vi "Scale Thumb.vi"(2 "Desired Dimensions":cluster{"Width":i32, "Height":i32}={"Width"=-1, "Height"=-1}, 3 "Full Size":bool=TRUE, 4 "Offset":cluster{"X":sgl, sgl}={"X"=-1.0, 0.0}, 5 "file":string, 6 "picture in":picture, 7 "Mod":T1) -> (0 "frame":T2, 1 "new picture":picture)   [LabVIEW 2012]
uses:
  SlideParams.ctl
  LVPresent_Globals.vi
panel:
  out "Dimensions":cluster{"Width":i32, "Height":i32}
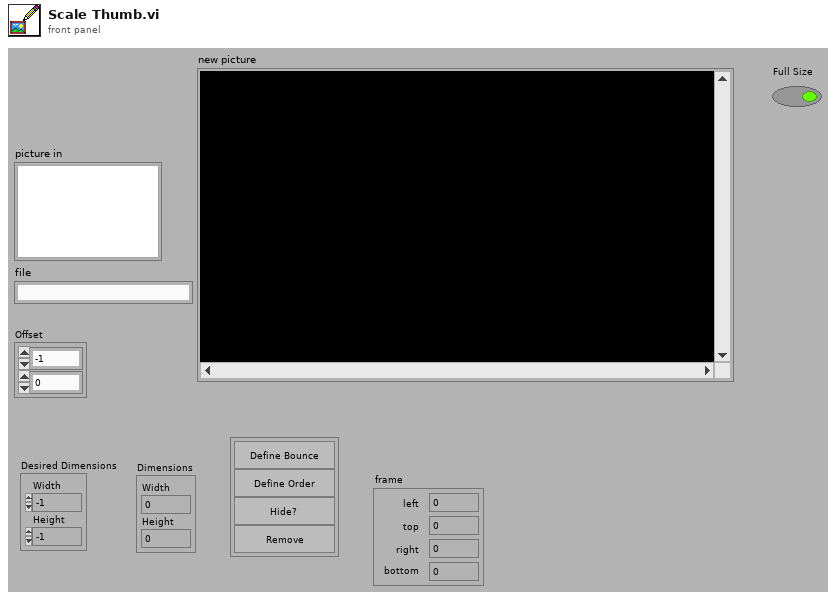
[diagram p1: front panel]
types:
  T1 = typedef "SlideParams.ctl" = enum32{"No Selection", "Bounce", "Order", "Hide", "Remove"}
  T2 = cluster{"left":i16, "top":i16, "right":i16, "bottom":i16}
  T3 = typedef "LVPositionTypeDef.ctl" = cluster{"Left":i32, "Top":i32}
  T4 = typedef "ParamterCluster.ctl" = cluster{"bounce?":bool, "black?":bool, "slide number":i32, "hide?":bool, "selection":bool}
  T5 = typedef "QT_Image.ctl" = cluster{"Width":i32, "Height":i32, "Depth":i32, "data":u8[], "Compressed data":u8[], "Color table":u32[], "Duration":i32, "Options":i32, "Timestamp":i32, "ID":i32, "Reserved":i32, "Dialogs":u32}
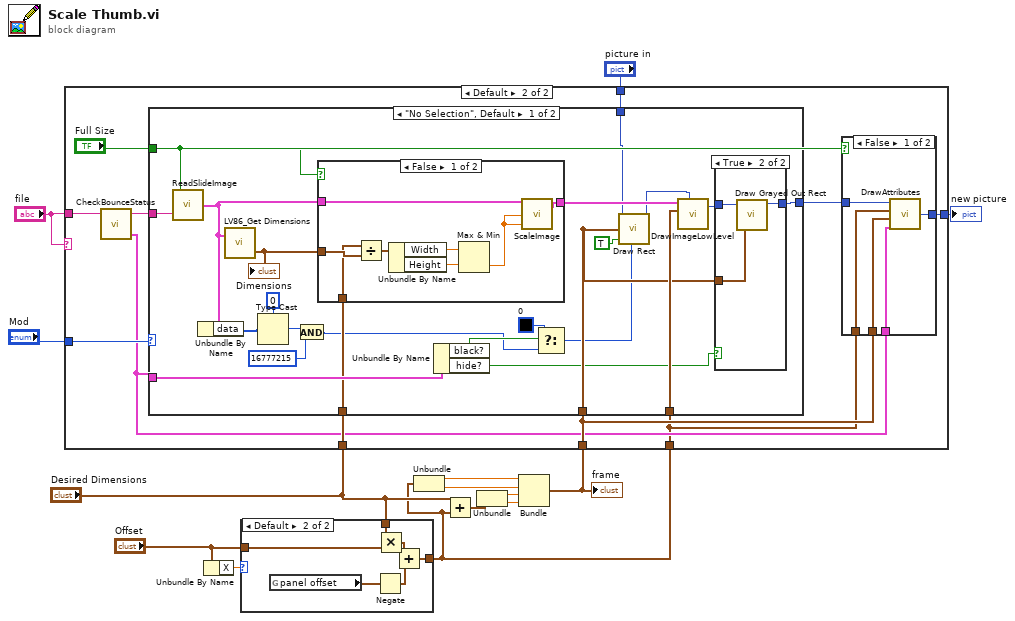
[diagram p0: block diagram]
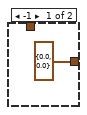
[diagram p2: hidden frame]
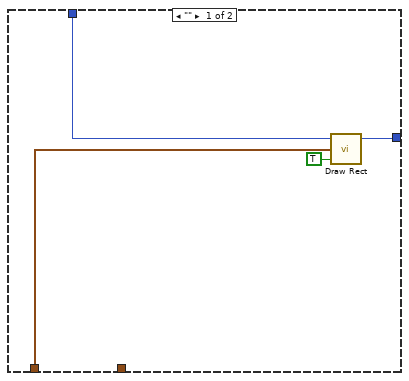
[diagram p3: hidden frame]
diagram:
  n1 = Unbundle By Name("Offset") -> ("X"=w1:sgl)
  n2 = case shown="Default" w1 {
    tunnel: "Desired Dimensions" -> [_ w20]
    tunnel: [cluster{sgl, sgl} {0.0, 0.0} w18] -> w3
    tunnel: "Offset" -> [_ w16]
    frame -1 {
    }
    frame Default {
      n3 = global read "LVPresent_Globals.vi" "panel offset"() -> (w17:T3)
      n4 = Negate(x=w17) -> (-x=w19:T3)
      n5 = Multiply(x=w20, y=w16) -> (x*y=w21:cluster{sgl, sgl})
      n6 = Add(x=w21, y=w19) -> (x+y=w18:cluster{sgl, sgl})
    }
  }
  n7 = Unbundle(w3) -> (w13:sgl, w12:sgl)
  n8 = Add(x="Desired Dimensions", y=w3) -> (x+y=w11:cluster{sgl, sgl})
  n9 = Unbundle(w11) -> (w10:sgl, w9:sgl)
  n10 = Bundle(w13, w12, w10, w9) -> (w7:cluster{sgl, sgl, sgl, sgl})  [unwired: 1 in]
  "frame" <- w7
  n11 = case shown="Default" "file" {
    tunnel: "picture in" -> [w25 w36]
    tunnel: "Desired Dimensions" -> [_ w35]
    tunnel: "file" -> [_ w33]
    tunnel: [w24 w31] -> w8
    tunnel: w7 -> [w23 w30]
    tunnel: w3 -> [_ w27]
    tunnel: "Mod" -> [_ w29]
    frame "" {
      n12 = call <vilib>:"Draw Rect.vi"("picture"=w25, "rect"=w23, "fill?(F)"=TRUE) -> ("new picture"=w24:picture)  [unwired: 6 in]
    }
    frame Default {
      n13 = call "CheckBounceStatus.vi"("File Name"=w33) -> ("Parameters"=w28:T4, "file name"=w34:string)  [unwired: 1 in, 1 out]
      n14 = case shown="\"No Selection\", Default" w29 {
        tunnel: w36 -> [w51 w79]
        tunnel: w35 -> [w55 _]
        tunnel: w34 -> [w54 _]
        tunnel: [w58 w79] -> w32
        tunnel: w30 -> [w59 _]
        tunnel: w27 -> [w63 _]
        tunnel: w28 -> [w62 _]
        tunnel: "Full Size" -> [w53 _]
        frame "No Selection", Default {
          n15 = call "ReadSlideImage.vi"("file name"=w54, "Full Size"=w53) -> ("Image"=w44:T5)
          n16 = Unbundle By Name(w44) -> ("data"=w45:u8[])
          n17 = call <userlib>:"LV86_Get Dimensions.vi"("Image In"=w44) -> ("Dimensions"=w56:cluster{"Width":i32, "Height":i32})  [unwired: 1 in, 1 out]
          "Dimensions" <- w56
          n18 = Type Cast(type=u32 0 ("index (row)"), x=w45) -> (*(type *) &x=w46:u32)
          n19 = And(x=w46, y=u32 16777215 ("hi")) -> (x .and. y?=w43:u32)
          n20 = case shown="False" w53 {
            tunnel: [w73 w74] -> w65
            tunnel: w44 -> [w72 w74]
            tunnel: w56 -> [w67 _]
            tunnel: w55 -> [w66 _]
            frame False {
              n21 = Divide(x=w66, y=w67) -> (x/y=w71:cluster{"Width":dbl, "Height":dbl})
              n22 = Unbundle By Name(w71) -> ("Width"=w69:dbl, "Height"=w70:dbl)
              n23 = Max & Min(x=w69, y=w70) -> (min(x,y)=w68:dbl)  [unwired: 1 out]
              n24 = call <userlib>:"ScaleImage.vi"("X scale"=w68, "Y scale"=w68, "Image in"=w72) -> ("Image Out"=w73:T5)  [unwired: 2 in]
            }
            frame True {
            }
          }
          n25 = Unbundle By Name(w62) -> ("black?"=w61:bool, "hide?"=w57:bool)
          n26 = Select(t=u32 0 ("color(black)"), s=w61, f=w43) -> (s? t:f=w49:u32)
          n27 = call <vilib>:"Draw Rect.vi"("picture"=w51, "rect"=w59, "fill?(F)"=TRUE, "color(black)"=w49) -> ("new picture"=w50:picture)  [unwired: 5 in]
          n28 = call <userlib>:"DrawImageLowLevel.vi"("Image"=w65, "Position"=w63, "picture in"=w50) -> ("new picture"=w52:picture)  [unwired: 2 in, 1 out]
          n29 = case shown="True" w57 {
            tunnel: w52 -> [w75 w78]
            tunnel: w59 -> [_ w77]
            tunnel: [w75 w76] -> w58
            frame False {
            }
            frame True {
              n30 = call <vilib>:"Draw Grayed Out Rect.vi"("rect"=w77, "picture"=w78) -> ("new picture"=w76:picture)  [unwired: 3 in]
            }
          }
        }
        frame "Bounce", "Order" {
        }
      }
      n31 = case shown="False" "Full Size" {
        tunnel: w32 -> [w41 w42]
        tunnel: [w40 w42] -> w31
        tunnel: w30 -> [w39 _]
        tunnel: w28 -> [w38 _]
        tunnel: w27 -> [w37 _]
        frame False {
          n32 = call "DrawAttributes.vi"("Parameters"=w38, "rect"=w39, "upper Left"=w37, "image in"=w41) -> ("image out"=w40:picture)
        }
        frame True {
        }
      }
    }
  }
  "new picture" <- w8
